vi "SnapShot_Video.vi"(8 "error in (no error)":errorcluster, 9 "Snnp Shot Path":path=path "C:/DeleteMe/test.png", 11 "VLC Variables":T1) -> (0 "error out":errorcluster, 3 "VLC Variables Out":T1)   [LabVIEW 2012]
uses:
  Controls-Webcam/VLC Var.ctl
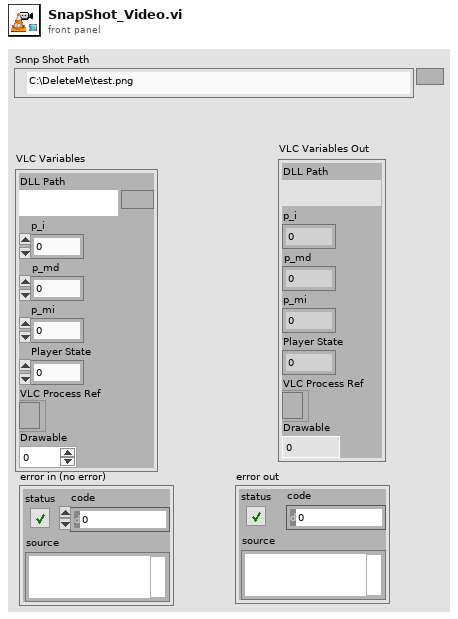
[diagram p1: front panel]
types:
  T1 = typedef "VLC Var.ctl" = cluster{"DLL Path":path, "p_i":i32, "p_md":i32, "p_mi":i32, "Player State":i32, "VLC Process Ref":refnum<k24>, "Drawable":i32}
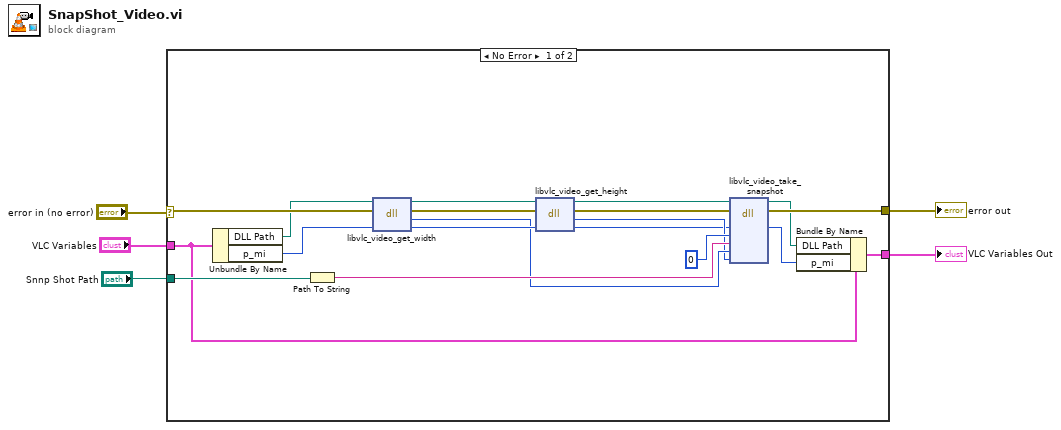
[diagram p0: block diagram]
diagram:
  n1 = case shown="No Error" "error in (no error)" {
    selector: "error in (no error)" -> [w11 w26]
    tunnel: "VLC Variables" -> [w10 w25]
    tunnel: [w14 w26] -> w4
    tunnel: "Snnp Shot Path" -> [w12 _]
    tunnel: [w8 w25] -> w1
    frame No Error {
      n2 = Unbundle By Name(w10) -> ("DLL Path"=w6:path, "p_mi"=w13:i32)
      n3 = Path To String(path=w12) -> (string=w24:string)
      n4 = dll-call lib="C:/Program Files/VideoLAN/VLC/libvlc.dll" fn="libvlc_video_get_width"(path in=w6, error in=w11, "p_mi"=w13) -> (path out=w20:path, error out=w21:errorcluster, "return type"=w19:i32, "p_mi"=w22:i32)  [unwired: 1 in]
      n5 = dll-call lib="C:/Program Files/VideoLAN/VLC/libvlc.dll" fn="libvlc_video_get_height"(path in=w20, error in=w21, "p_mi"=w22) -> (path out=w16:path, error out=w17:errorcluster, "return type"=w18:i32, "p_mi"=w15:i32)  [unwired: 1 in]
      n6 = dll-call lib="C:/Program Files/VideoLAN/VLC/libvlc.dll" fn="libvlc_video_take_snapshot"(path in=w16, error in=w17, "p_mi"=w15, "unsigned_num"=u32 0, "psz_filepath"=w24, "i_width"=w19, "i_height"=w18) -> (path out=w7:path, error out=w14:errorcluster, "p_mi"=w9:i32)  [unwired: 6 in]
      n7 = Bundle By Name(cluster=w10, "DLL Path"=w7, "p_mi"=w9) -> (w8:T1)
    }
    frame Error {
    }
  }
  "error out" <- w4
  "VLC Variables Out" <- w1
